vi "RecordAPP.vi"() -> ()   [LabVIEW 2022 SP3]
uses:
  <vilib>/sound2/lvsound2.llb/Sound Data Format.ctl
  <vilib>/sound2/lvsound2.llb/Sound Input Task ID.ctl
  <vilib>/Utility/miscctls.llb/LVPointTypeDef.ctl
  <vilib>/sound2/lvsound2.llb/Sound Input Read (DBL).vi
  <vilib>/sound2/lvsound2.llb/Sound Output Write (DBL Single).vi
  <vilib>/regexp/Match Regular Expression.xnode
  <vilib>/sound2/lvsound2.llb/Sound Output Write (DBL).vi
panel:
  in  "expand":bool
  out "Record":bool
  out "Play":bool
  in  "Sec.Play(K)":bool
  out "Resolution":dbl format="%.10f"
  out "Record_Graph":cluster{"x":dbl[], "y":dbl[]}(graph)
  in  "device ID":u32
  out "Record":waveform(dbl)[](graph)
  in  "stop":bool
  out "error out":errorcluster
  in  "AnalysisRecord_read(M)":bool
  in  "StartStopRecord(B)":bool
  in  "path":path
  out "VoiceData":dbl[](array[numeric])
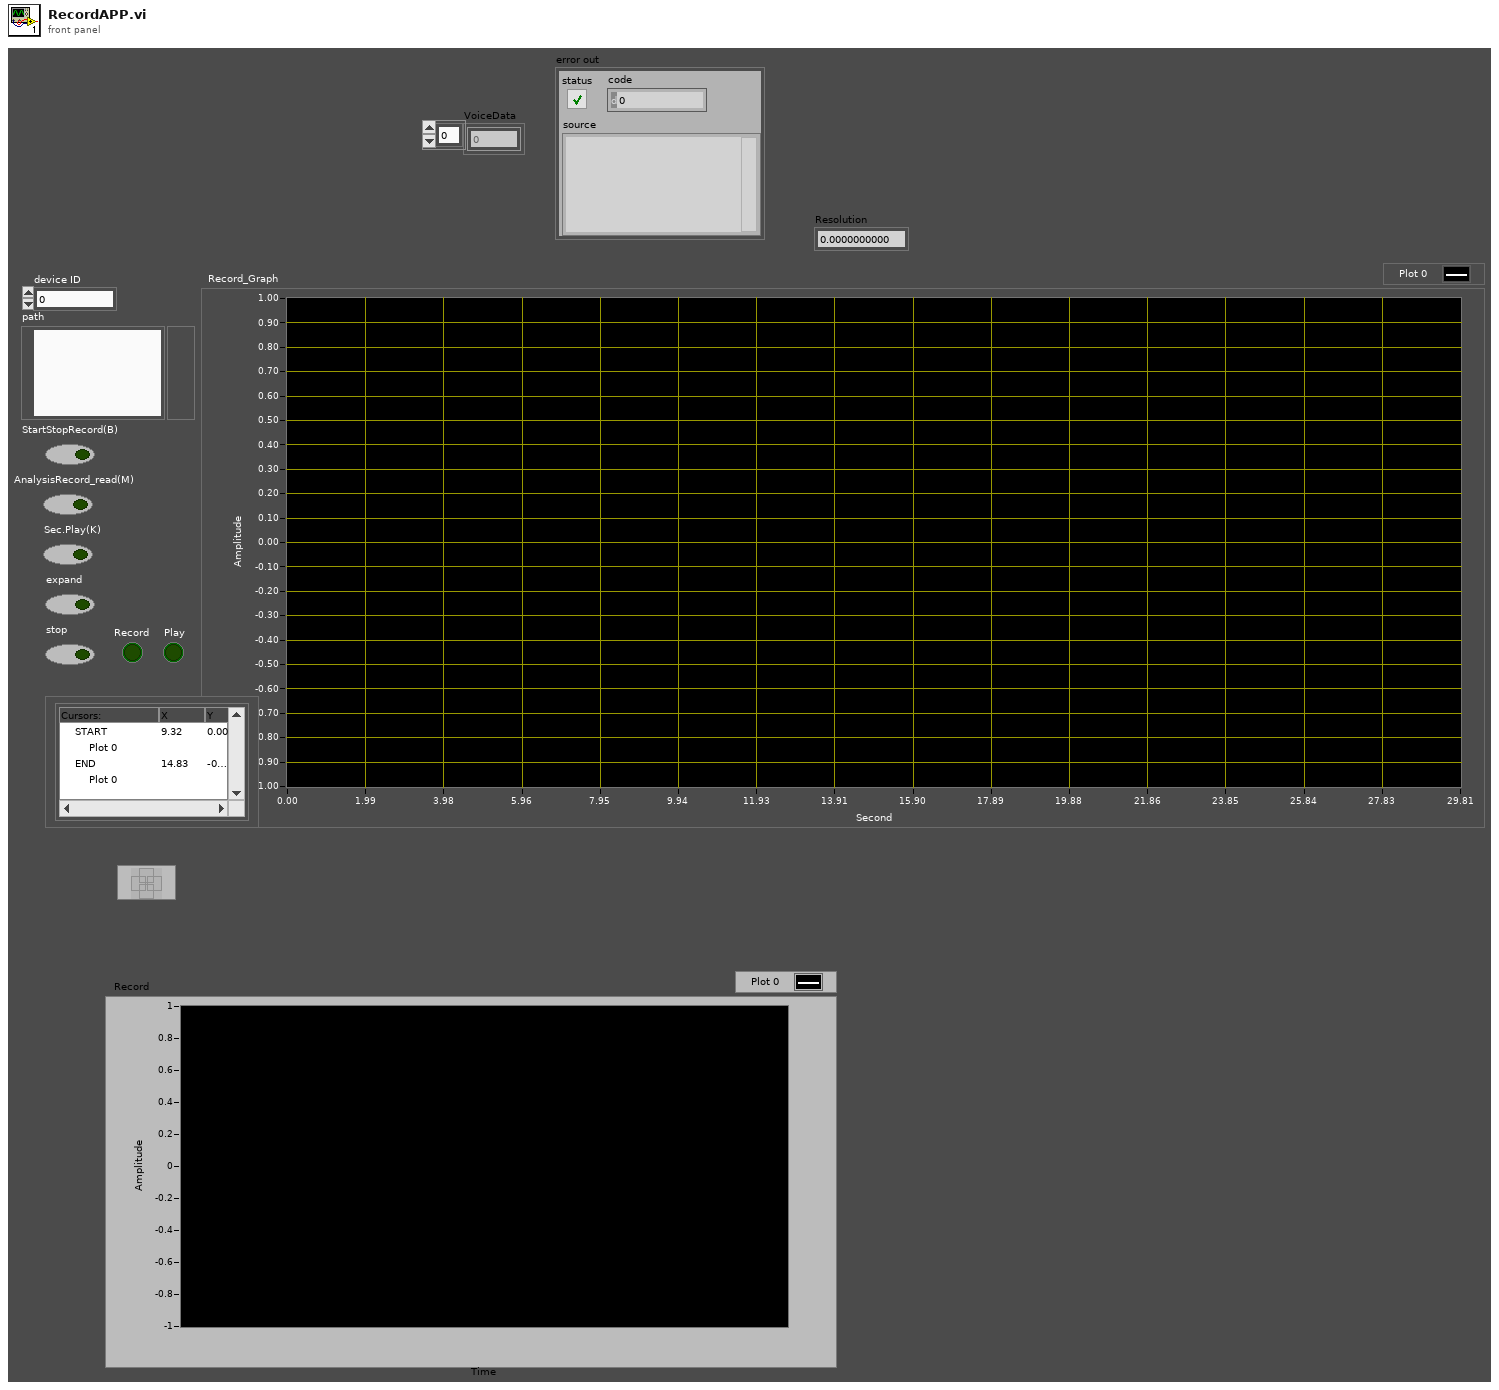
[diagram p1: front panel]
types:
  T1 = typedef "Sound Data Format.ctl" = cluster{"sample rate (S/s)":dbl, "number of channels":i32, "bits per sample":i32}
  T2 = typedef "LVPointTypeDef.ctl" = cluster{"Horizontal":i16, "Vertical":i16}
  T3 = typedef "Sound Input Task ID.ctl" = u32
  T4 = typedef "LVRectTypeDef.ctl" = cluster{"Left":i16, "Top":i16, "Right":i16, "Bottom":i16}
  T5 = typedef "Sound Output Task ID.ctl" = u32
  T6 = enum16{"open", "open or create", "create or replace", "create", "open (read-only)"}
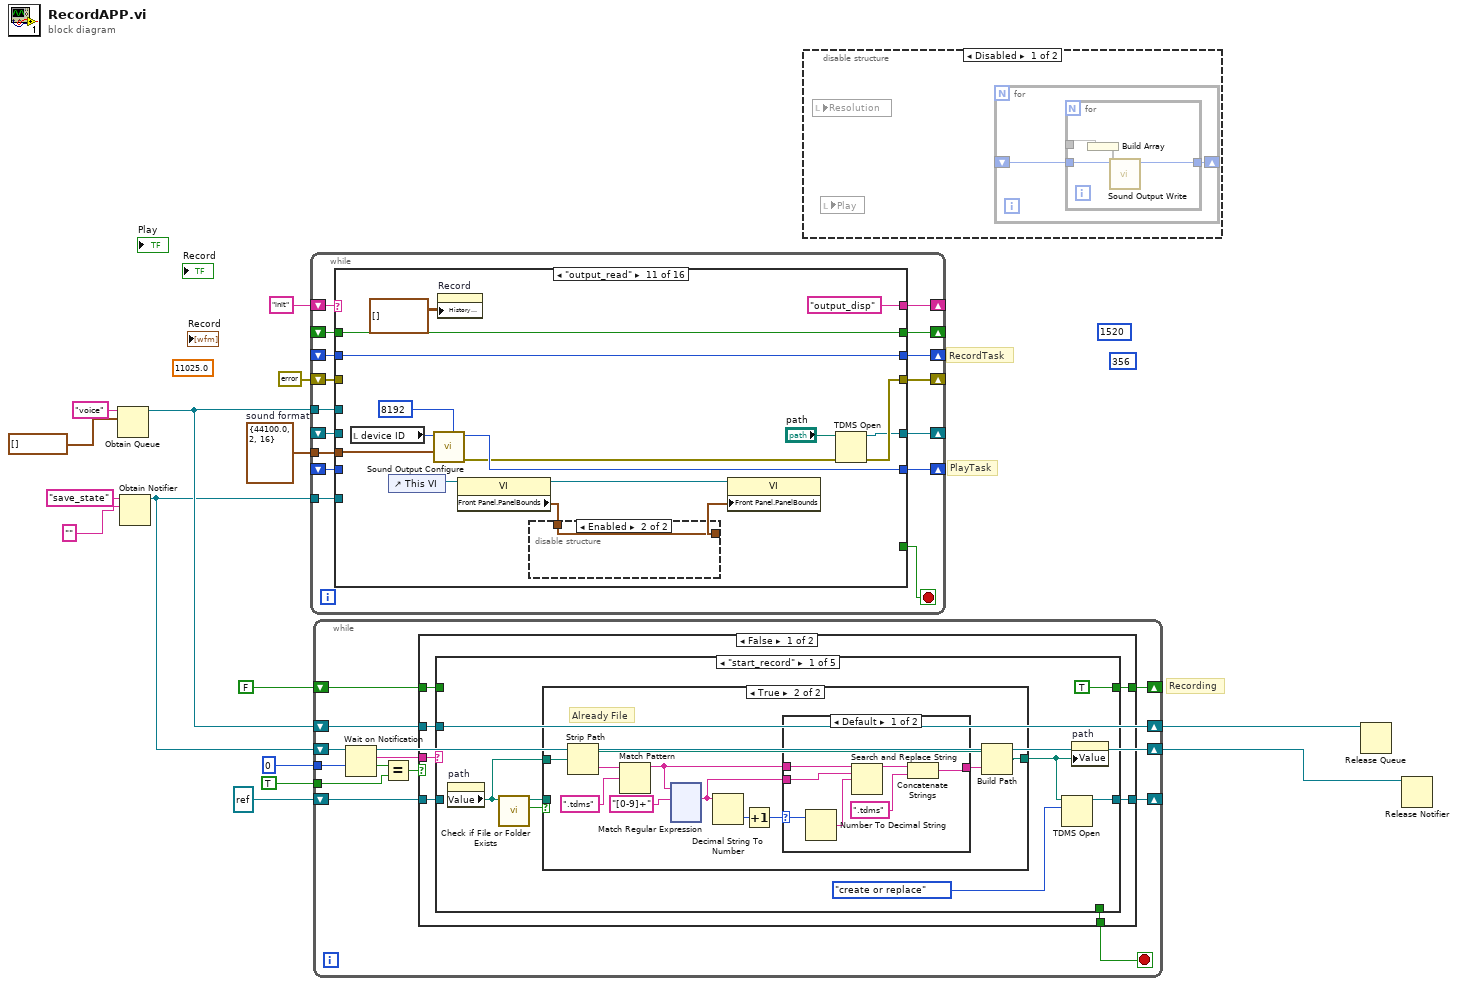
[diagram p0: block diagram]
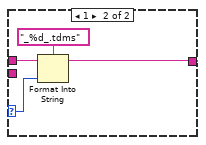
[diagram p4: hidden frame]
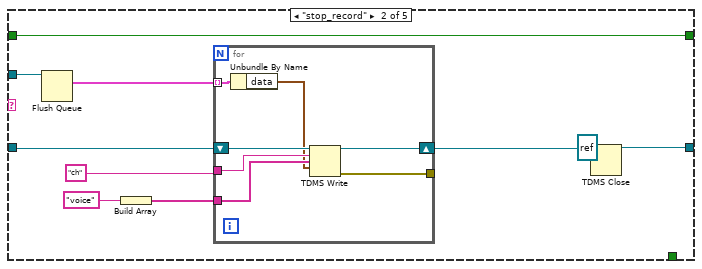
[diagram p5: hidden frame]
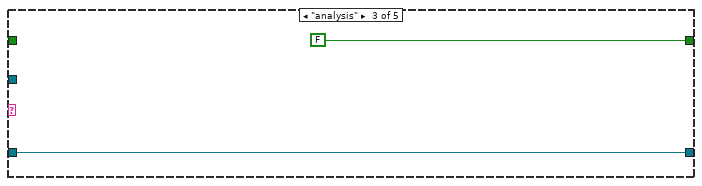
[diagram p6: hidden frame]
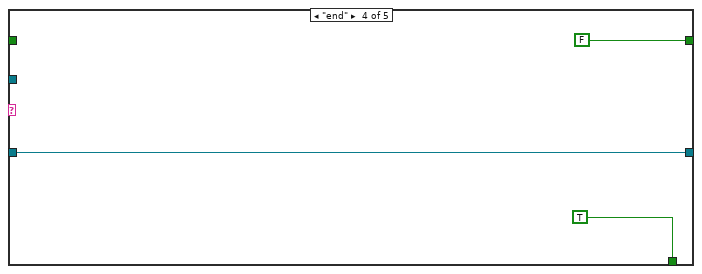
[diagram p7: hidden frame]
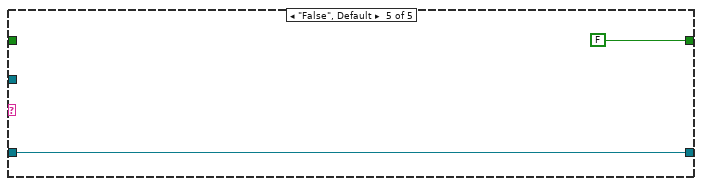
[diagram p8: hidden frame]
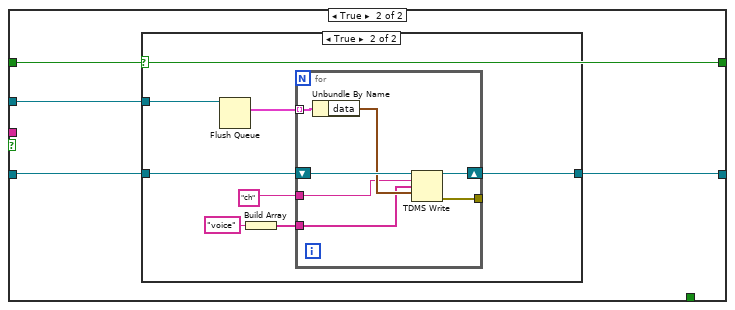
[diagram p9: hidden frame]
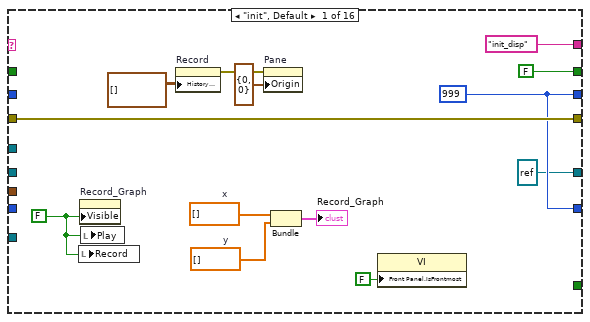
[diagram p11: hidden frame]
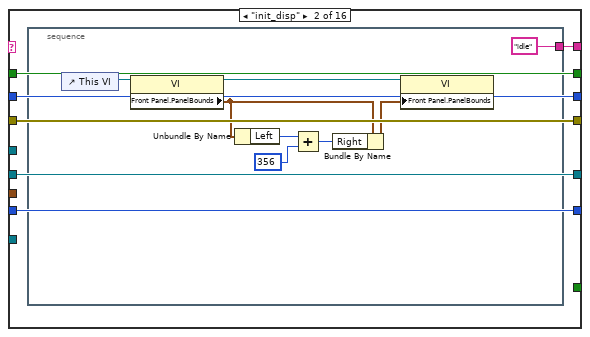
[diagram p12: hidden frame]
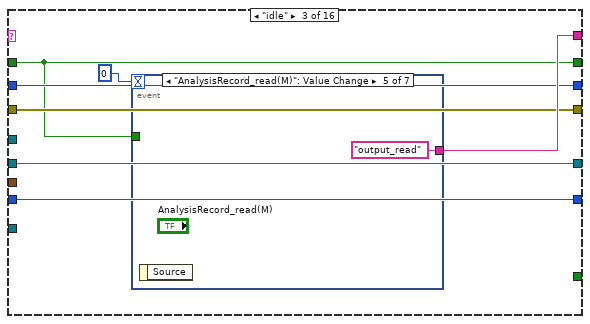
[diagram p13: hidden frame]
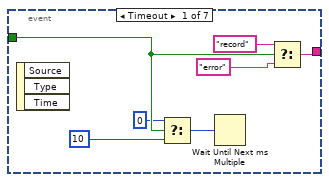
[diagram p14: hidden frame]
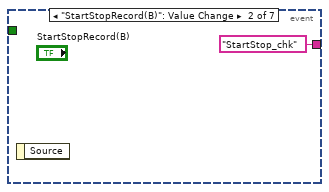
[diagram p15: hidden frame]
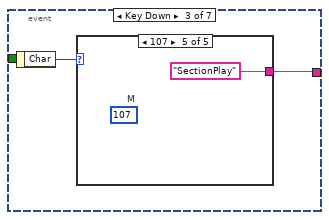
[diagram p16: hidden frame]
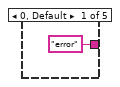
[diagram p17: hidden frame]
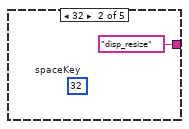
[diagram p18: hidden frame]
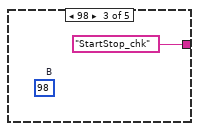
[diagram p19: hidden frame]
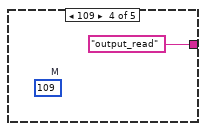
[diagram p20: hidden frame]
diagram:
  (unwired) u32 356 ("Bounds:Area Width 2")
  (unwired) u32 1520 ("Bounds:Area Width")
  (unwired) 11025.0 ("sample rate (S/s)")
  w2 = T1 {"sample rate (S/s)"=44100.0, "number of channels"=2, "bits per sample"=16}  # sound format
  # "Recording"
  # "RecordTask"
  # "PlayTask"
  n1 = Obtain Queue(name (unnamed)="voice", element data type=waveform(dbl)[] [] ("data")) -> (queue out=w11:refnum<queue>)  [unwired: 3 in, 2 out]
  n2 = Obtain Notifier(name (unnamed)="save_state", notification data type="") -> (notifier out=w7:refnum<notifier>)  [unwired: 2 in, 2 out]
  n3 = while {
    shift-right: [w30] -> _
    shift-left: "init" -> [w31]
    shift-right: [w29] -> _
    shift-left: _ -> [w28]
    shift-right: [w27] -> _
    shift-left: errorcluster {"status"=FALSE, "code"=0, "source"=""} ("error out") -> [w26]
    shift-right: [w25] -> _
    shift-left: _ -> [w24]
    tunnel: w11 -> [w23]
    tunnel: w7 -> [w22]
    tunnel: w2 -> [w20]
    shift-right: [w19] -> _
    shift-left: _ -> [w18]
    shift-right: [w17] -> _
    shift-left: _ -> [w16]
    stop <- w21 stop-if-true
    n4 = case shown="\"output_read\"" w31 {
      tunnel: ["init_disp" w50 w64 w98 w107 w114 w133 "error" "idle" "idle" "output_disp" "output_disp2" w240 w293 "idle" "end"] -> w30
      tunnel: [w40 w49 w63 w100 w106 w113 w132 w157 w173 T3 999 ("task ID out") w204 w233 w239 w292 w323 w332] -> w29
      tunnel: w28 -> [_ w49 w63 w100 w106 w113 w132 _ w172 w188 w204 w233 w239 w292 w323 w332]
      tunnel: [w43 w48 w62 w96 w105 w112 w131 w156 w162 w176 w201 w232 w238 w291 w320 w331] -> w27
      tunnel: w26 -> [w43 w48 w62 w96 w105 w112 w131 w147 w171 w185 _ w232 w238 w291 w322 w331]
      tunnel: [FALSE w47 w61 w95 w104 w111 w130 TRUE w174 FALSE w203 w231 w237 w290 w321 w330] -> w25
      tunnel: w24 -> [_ w47 w61 w95 w104 w111 w130 _ w174 _ w203 w231 w237 w290 w321 w330]
      tunnel: w23 -> [_ _ _ _ _ _ _ _ w170 _ _ _ _ _ _ _]
      tunnel: w22 -> [_ _ _ _ _ _ _ w153 _ w181 _ w224 _ _ _ w328]
      tunnel: [_ _ _ _ _ _ _ _ _ _ _ _ _ _ _ TRUE] -> w21
      tunnel: w20 -> [_ _ _ _ _ _ _ w158 _ _ w198 _ _ _ _ _]
      tunnel: [refnum<k34> refnum ("tdms file out") w46 w60 w93 w103 w110 w129 w151 w166 w180 w200 refnum<k34> refnum ("tdms file out") w236 w289 w319 w326] -> w19
      tunnel: w18 -> [_ w46 w60 w93 w103 w110 w129 w151 w166 w180 _ w230 w236 w289 w319 w326]
      tunnel: [w40 w45 w59 w92 w102 w109 w128 w150 w165 w179 w196 w217 w235 w287 w318 w325] -> w17
      tunnel: w16 -> [_ w45 w59 w92 w102 w109 w128 w150 w165 w179 _ w217 w235 w288 w318 w325]
      frame "init", Default {
        w35 = dbl[] []  # y
        w36 = dbl[] []  # x
        w38 = FALSE ("Visible")
        w40 = T3 999 ("task ID out")
        n5 = local write "Record"(w38) -> ()
        n6 = property on="Record_Graph" class="XYGraph (strict)"("Visible"=w38) -> ()  [unwired: 2 in, 2 out]
        n7 = local write "Play"(w38) -> ()
        n8 = property on="Record" class="WFChart (strict)"("History Data"=waveform(dbl)[][] []) -> (error out=w34:errorcluster)  [unwired: 2 in, 1 out]
        n9 = property on="Pane" class="Pane"(error in=w34, "Origin"=T2 {"Horizontal"=0, "Vertical"=0}) -> ()  [unwired: 1 in, 2 out]
        n10 = Bundle("x"=w36, "y"=w35) -> (→"Record_Graph":cluster{"x":dbl[], "y":dbl[]})  [unwired: 1 in]
        n11 = property class="VI"("Front Panel.IsFrontmost"=FALSE ("Front Panel Window:Is Frontmost")) -> ()  [unwired: 2 in, 2 out]
      }
      frame "init_disp" {
        n12 = stacked-sequence {
          tunnel: ["idle"] -> w50
          frame #0 {
            n13 = control-ref of="This VI"() -> (w57:refnum<vi>)
            n14 = property class="VI"(reference=w57) -> (reference out=w56:refnum<vi>, "Front Panel.PanelBounds"=w53:T4)  [unwired: 1 in, 1 out]
            n15 = Unbundle By Name(w53) -> ("Left"=w55:i16)
            n16 = Add(x=w55, y=u32 356 ("Bounds:Area Width 2")) -> (x+y=w51:u32)
            n17 = Bundle By Name(cluster=w53, "Right"=w51) -> (w52:T4)
            n18 = property class="VI"(reference=w56, "Front Panel.PanelBounds"=w52) -> ()  [unwired: 1 in, 2 out]
          }
        }
      }
      frame "idle" {
        n19 = event shown="[4] \"AnalysisRecord_read(M)\": Value Change" {
          selector: _ -> [_ _ _ _ _ _ _]
          dyn-events: _ -> [_ _ _ _ _ _ _]
          timeout: 0 -> [_ _ _ _ _ _ _]
          tunnel: [w71 "StartStop_chk" w74 "end" "output_read" ("t") "SectionPlay" ("t") "expand" ("t")] -> w64
          tunnel: w61 -> [w68 _ _ _ _ _ _]
          event Timeout {
            n20 = event-data() -> ()  [unwired: 1 in, 3 out]
            n21 = Select(t=u32 0, s=w68, f=u32 10 ("millisecond multiple")) -> (s? t:f=w69:u32)
            n22 = Wait Until Next ms Multiple(millisecond multiple=w69) -> ()  [unwired: 1 out]
            n23 = Select(t="record", s=w68, f="error") -> (s? t:f=w71:string)
          }
          event "StartStopRecord(B)": Value Change {
            n24 = event-data() -> ()  [unwired: 1 in, 1 out]
          }
          event Key Down {
            n25 = event-data() -> ("Char"=w75:i16)  [unwired: 1 in]
            n26 = case shown="107" w75 {
              tunnel: ["error" ("t") "disp_resize" ("t") "StartStop_chk" ("t") "output_read" ("t") "SectionPlay" ("t")] -> w74
              frame 0, Default {
              }
              frame 32 {
                (unwired) i16 32  # spaceKey
              }
              frame 98 {
                (unwired) i16 98  # B
              }
              frame 109 {
                (unwired) i16 109  # M
              }
              frame 107 {
                (unwired) i16 107  # M
              }
            }
          }
          event "stop": Value Change {
            n27 = event-data() -> ()  [unwired: 1 in, 1 out]
          }
          event "AnalysisRecord_read(M)": Value Change {
            n28 = event-data() -> ()  [unwired: 1 in, 1 out]
          }
          event "Sec.Play(K)": Value Change {
            n29 = event-data() -> ()  [unwired: 1 in, 1 out]
          }
          event "expand": Value Change {
            n30 = event-data() -> ()  [unwired: 1 in, 1 out]
          }
        }
      }
      frame "StartStop_chk" {
        n31 = control-ref of="This VI"() -> (w91:refnum<vi>)
        n32 = Equal?(x=w100, y=T3 999) -> (x = y?=w94:bool)
        n33 = property class="VI"(reference=w91) -> (reference out=w90:refnum<vi>, "Front Panel.PanelBounds"=w87:T4)  [unwired: 1 in, 1 out]
        n34 = Unbundle By Name(w87) -> ("Left"=w89:i16)
        n35 = Add(x=w89, y=u32 356 ("Bounds:Area Width 2")) -> (x+y=w85:u32)
        n36 = Bundle By Name(cluster=w87, "Right"=w85) -> (w86:T4)
        n37 = property class="VI"(reference=w90, "Front Panel.PanelBounds"=w86) -> ()  [unwired: 1 in, 2 out]
        n38 = Select(t="start", s=w94, f="stop") -> (s? t:f=w98:string)
      }
      frame "xxxxxxxxxxx" {
        n39 = stacked-sequence {
          tunnel: ["idle"] -> w107
          frame #0 {
          }
        }
      }
      frame "disp_resize" {
        n40 = stacked-sequence {
          tunnel: ["idle"] -> w114
          frame #0 {
            w117 = u32 356 ("Bounds:Area Width 2")
            n41 = property class="VI"() -> (reference out=w126:refnum<vi>, "Front Panel.PanelBounds"=w125:T4)  [unwired: 2 in, 1 out]
            n42 = Unbundle By Name(w125) -> ("Right"=w123:i16, "Left"=w118:i16)
            n43 = Subtract(x=w123, y=w118) -> (x-y=w122:i16)
            n44 = Less Or Equal?(x=w122, y=w117) -> (x <= y?=w120:bool)
            n45 = Add(x=w118, y=w117) -> (x+y=w116:u32)
            n46 = Add(x=w118, y=u32 1520 ("Bounds:Area Width")) -> (x+y=w115:u32)
            n47 = Select(t=w115, s=w120, f=w116) -> (s? t:f=w121:u32)
            n48 = Bundle By Name(cluster=w125, "Right"=w121) -> (w124:T4)
            n49 = property class="VI"(reference=w126, "Front Panel.PanelBounds"=w124) -> ()  [unwired: 1 in, 2 out]
          }
        }
      }
      frame "expand" {
        n50 = stacked-sequence {
          tunnel: ["idle"] -> w133
          frame #0 {
            w140 = 10
            w141 = u32 1  # y
            w142 = u32 0  # x
            n51 = property on="Record_Graph" class="XYGraph (strict)"("Active Cursor"=w142, "Active Cursor"=w141) -> ("Cursor.Cursor X"=w135:dbl, "Cursor.Cursor X"=w136:dbl)  [unwired: 2 in, 2 out]
            n52 = Subtract(x=w136, y=w135) -> (x-y=w134:dbl)
            n53 = Divide(x=w134, y=w140) -> (x/y=w139:dbl)
            n54 = for {
              N: w140 -> [_]
              tunnel: w139 -> [w146]
              tunnel: [w144] -> w138 mode=indexing
              shift-right: [w144] -> _
              shift-left: w135 -> [w145]
              n55 = Add(x=w145, y=w146) -> (x+y=w144:dbl)
            }
            n56 = Build Array (concatenate)(w135, w138) -> (w137:dbl[])
            n57 = property on="Record_Graph" class="XYGraph (strict)"("XScale.RngStart"=w135, "XScale.Minimum"=w135, "XScale.Maximum"=w136, "XScale.Increment"=w139, "XScale.MarkerVals[]"=w137) -> ()  [unwired: 2 in, 2 out]
          }
        }
      }
      frame "start" {
        n58 = property on="Record_Graph" class="XYGraph (strict)"("Visible"=FALSE) -> ()  [unwired: 2 in, 2 out]
        n59 = local write "Record"(TRUE ("Record")) -> ()
        n60 = Send Notification(notification="start_record", notifier=w153, error in (no error)=w147) -> (error out=w152:errorcluster)  [unwired: 1 out]
        n61 = call <vilib>:"Sound Input Configure.vi"("number of samples/ch"=8192, "error in (no error)"=w152, "sound format"=w158, "device ID"="device ID") -> ("error out"=w156:errorcluster, "task ID"=w157:T3)  [unwired: 6 in]
      }
      frame "record" {
        n62 = Quotient & Remainder(x=8192 ("number of samples/ch"), y=2) -> (floor(x/y)=w167:i32)  [unwired: 1 out]
        n63 = call-poly <vilib>:"Sound Input Read.vi"("number of samples/ch"=w167, "error in (no error)"=w171, "task ID"=w172) -> ("error out"=w163:errorcluster, "data"=w164:waveform(dbl)[], "task ID out"=w173:T3)  [unwired: 6 in]
        n64 = Enqueue Element(queue=w170, element=w164, error in (no error)=w163) -> (error out=w162:errorcluster)  [unwired: 1 in, 2 out]
      }
      frame "stop" {
        n65 = call <vilib>:"Sound Input Stop.vi"("error in (no error)"=w185, "task ID"=w188) -> ("error out"=w186:errorcluster, "task ID out"=w187:T3)  [unwired: 8 in]
        n66 = call <vilib>:"Sound Input Clear.vi"("error in (no error)"=w186, "task ID"=w187) -> ("error out"=w182:errorcluster)  [unwired: 9 in]
        n67 = Send Notification(notification="stop_record", notifier=w181, error in (no error)=w182) -> (error out=w176:errorcluster)  [unwired: 1 out]
        n68 = local write "Record"(FALSE ("Record")) -> ()
      }
      frame "output_read" {
        n69 = local read "device ID"() -> (w199:u32)
        n70 = control-ref of="This VI"() -> (w193:refnum<vi>)
        n71 = call <vilib>:"Sound Output Configure.vi"("number of samples/ch"=8192, "sound format"=w198, "device ID"=w199) -> ("error out"=w194:errorcluster, "task ID"=w196:T5)  [unwired: 7 in]
        n72 = property on="Record" class="WFChart (strict)"("History Data"=waveform(dbl)[][] []) -> ()  [unwired: 2 in, 2 out]
        n73 = property class="VI"(reference=w193) -> (reference out=w192:refnum<vi>, "Front Panel.PanelBounds"=w191:T4)  [unwired: 1 in, 1 out]
        n74 = disable-structure shown="Enabled" {
          disable-tunnel: w191 -> [w209 w211]
          disable-tunnel: [w208 w211] -> w190
          frame Disabled {
            n75 = Unbundle By Name(w209) -> ("Left"=w210:i16)
            n76 = Add(x=w210, y=u32 1520 ("Bounds:Area Width")) -> (x+y=w207:u32)
            n77 = Bundle By Name(cluster=w209, "Right"=w207) -> (w208:T4)
          }
          frame Enabled {
          }
        }
        n78 = property class="VI"(reference=w192, "Front Panel.PanelBounds"=w190) -> ()  [unwired: 1 in, 2 out]
        n79 = TDMS Open(8:w194, 11:"path") -> (0:w201:errorcluster, 3:w200:refnum<k34>)  [unwired: 5 in]
      }
      frame "output_disp" {
        w215 = "voice" ("group name in")
        n80 = Build Array(w215) -> (w227:string[])
        n81 = TDMS Read(0:w230, 5:"ch" ("group name in"), 7:w227, 12:waveform(dbl)[] [] ("data")) -> (4:w221:refnum<k34>, 6:w216:string, 10:w226:waveform(dbl)[], 15:w223:errorcluster)  [unwired: 4 in, 2 out]
        n82 = Send Notification(notification="analysis", notifier=w224, error in (no error)=w223) -> (error out=w220:errorcluster)  [unwired: 1 out]
        n83 = local write "Record"(w226) -> ()
        n84 = TDMS Get Properties(5:0.0, 7:"wf_increment" ("channel name"), 8:w220, 9:w215, 10:w216, 11:w221) -> (0:w213:errorcluster, 3:w214:refnum<k34>, 4:→"Resolution":dbl)  [unwired: 3 out]
        n85 = TDMS Close(8:w213, 11:w214) -> ()  [unwired: 2 out]
      }
      frame "output_disp2" {
        n86 = stacked-sequence {
          seq-local: [_ w243 _ _] -> [_ _ w256 w273]
          seq-local: [_ w242 _ _] -> [_ _ _ w275]
          tunnel: [_ "idle" _ _] -> w240
          frame #0 {
            n87 = property on="Record_Graph" class="XYGraph (strict)"("Visible"=TRUE) -> ()  [unwired: 2 in, 2 out]
          }
          frame #1 {
            n88 = local read "Record"() -> (w248:waveform(dbl)[])
            n89 = local read "Resolution"() -> (w246:dbl)
            n90 = for {
              tunnel: w248 -> [w254] mode=indexing
              tunnel: [w253] -> w242 mode=concatenating
              n91 = Unbundle By Name(w254) -> ("Y"=w253:dbl[])
            }
            "VoiceData" <- w242
            n92 = Array Size(array=w242) -> (size(s)=w244:i32)
            n93 = for {
              N: w244 -> [_]
              tunnel: w246 -> [w252]
              tunnel: [w250] -> w243 mode=indexing
              i -> [w251]
              n94 = Multiply(x=w252, y=w251) -> (x*y=w250:dbl)
            }
            n95 = Bundle By Name(cluster=cluster{"x":dbl[], "y":dbl[]} {"x"=[], "y"=[]} ("output cluster"), "x"=w243, "y"=w242) -> (w245:cluster{"x":dbl[], "y":dbl[]})
            n96 = local write "Record_Graph"(w245) -> ()
          }
          frame #2 {
            w260 = 15
            n97 = Array Size(array=w256) -> (size(s)=w258:i32)
            n98 = Decrement(x=w258) -> (x-1=w255:i32)
            n99 = Index Array(array=w256, index #2=w255) -> (element #1=w259:dbl, element #2=w257:dbl)  [unwired: 1 in]
            n100 = Subtract(x=w257, y=w259) -> (x-y=w261:dbl)
            n101 = Divide(x=w261, y=w260) -> (x/y=w264:dbl)
            n102 = for {
              N: w260 -> [_]
              tunnel: w264 -> [w267]
              tunnel: [w265] -> w263 mode=indexing
              shift-right: [w265] -> _
              shift-left: w259 -> [w266]
              n103 = Add(x=w266, y=w267) -> (x+y=w265:dbl)
            }
            n104 = Build Array (concatenate)(w259, w263) -> (w262:dbl[])
            n105 = property on="Record_Graph" class="XYGraph (strict)"("XScale.RngStart"=w259, "XScale.Minimum"=w259, "XScale.Maximum"=w257, "XScale.Increment"=w264, "XScale.MarkerVals[]"=w262) -> ()  [unwired: 2 in, 2 out]
          }
          frame #3 {
            w282 = 0.5  # sec
            w286 = 0.5  # Hz
            n106 = Greater Or Equal?(x=w275, y=w286) -> (x >= y?=w285:bool[])
            n107 = Search 1D Array(1D array=w285, element=TRUE) -> (index of element=w283:i32)  [unwired: 1 in]
            n108 = Index Array(array=w273, index=w283) -> (element=w281:dbl)
            n109 = Subtract(x=w281, y=w282) -> (x-y=w280:dbl)
            n110 = Array Size(array=w273) -> (size(s)=w272:i32)
            n111 = Greater Or Equal?(x=w273, y=w280) -> (x >= y?=w278:bool[])
            n112 = Search 1D Array(1D array=w278, element=TRUE) -> (index of element=w270:i32)  [unwired: 1 in]
            n113 = Subtract(x=w272, y=500 ("x")) -> (x-y=w271:i32)
            n114 = Index Array(array=w273, index #1=w271, index #2=w270) -> (element #1=w276:dbl, element #2=w269:dbl)
            n115 = property on="Record_Graph" class="XYGraph (strict)"("Active Cursor"=u32 1, "Cursor.Cursor X"=w276, "Active Cursor"=u32 0, "Cursor.Cursor X"=w269) -> ()  [unwired: 2 in, 2 out]
          }
        }
      }
      frame "SectionPlay" {
        n116 = stacked-sequence {
          tunnel: [_ "idle" _] -> w293
          tunnel: w288 -> [_ w299 _]
          tunnel: [_ w297 _] -> w287
          frame #0 {
            n117 = local write "Play"(TRUE ("Play")) -> ()
          }
          frame #1 {
            w307 = u32 1  # y
            w308 = u32 0  # x
            n118 = local read "Record_Graph"() -> (w309:cluster{"x":dbl[], "y":dbl[]})
            n119 = property on="Record_Graph" class="XYGraph (strict)"("Active Cursor"=w308, "Active Cursor"=w307) -> ("Cursor.Cursor X"=w306:dbl, "Cursor.Cursor X"=w304:dbl)  [unwired: 2 in, 2 out]
            n120 = Unbundle By Name(w309) -> ("y"=w303:dbl[], "x"=w305:dbl[])
            n121 = Search 1D Array(1D array=w305, element=w306) -> (index of element=w301:i32)  [unwired: 1 in]
            n122 = Search 1D Array(1D array=w305, element=w304) -> (index of element=w302:i32)  [unwired: 1 in]
            n123 = Subtract(x=w302, y=w301) -> (x-y=w300:i32)
            n124 = Array Subset(array=w303, index=w301, length=w300) -> (w296:dbl[])
            n125 = for {
              N: 1 -> [_]
              tunnel: w299 -> [w315]
              tunnel: [w314] -> w297
              shift-right: [w312] -> _
              shift-left: dbl[] [0.0] -> [w312]
              tunnel: w296 -> [w311]
              tunnel: [w313] -> _
              n126 = Replace Array Subset(array=w312, new element=w312) -> ()  [unwired: 1 in, 1 out]
              n127 = call-poly <vilib>:"Sound Output Write.vi"("data"=w311, "task ID"=w315) -> ("error out"=w313:errorcluster, "task ID out"=w314:T5)  [unwired: 8 in]
            }
          }
          frame #2 {
            n128 = flat-sequence {
              frame #0 {
                n129 = Wait (ms)(milliseconds to wait=u32 50) -> ()  [unwired: 1 out]
              }
              frame #1 {
                n130 = local write "Play"(FALSE ("Play")) -> ()
              }
            }
          }
        }
      }
      frame "error" {
        n131 = call <vilib>:"Clear Errors.vi"("error in (no error)"=w322) -> ("error out"=w320:errorcluster)  [unwired: 5 in, 1 out]
        "error out" <- w322
      }
      frame "end" {
        n132 = Send Notification(notification="end", notifier=w328) -> ()  [unwired: 1 in, 2 out]
      }
    }
  }
  n133 = while {
    shift-right: [w341] -> _
    shift-left: FALSE -> [w340]
    tunnel: TRUE ("y") -> [w344]
    shift-right: [w339] -> _
    shift-left: refnum<k34> refnum ("tdms file out") -> [w337]
    shift-right: [w335] -> w4
    shift-left: w11 -> [w335]
    shift-right: [w336] -> w3
    shift-left: w7 -> [w346]
    tunnel: 0 ("timeout in ms (-1)") -> [w334]
    stop <- w338 stop-if-true
    n134 = Wait on Notification(notifier=w346, timeout in ms (-1)=w334) -> (notifier out=w336:refnum<notifier>, notification=w342:string, timed out?=w345:bool)  [unwired: 2 in, 1 out]
    n135 = Equal?(x=w345, y=w344) -> (x = y?=w343:bool)
    n136 = case shown="False" w343 {
      tunnel: w335 -> [w348 w526]
      tunnel: w342 -> [w353 _]
      tunnel: [w352 w527] -> w341
      tunnel: w340 -> [w351 w527]
      tunnel: [w350 w524] -> w339
      tunnel: w337 -> [w349 w525]
      tunnel: [w347 _] -> w338
      frame False {
        n137 = case shown="\"start_record\"" w353 {
          tunnel: [TRUE w509 FALSE FALSE FALSE] -> w352
          tunnel: w351 -> [_ w509 _ _ _]
          tunnel: [w358 refnum<k34> refnum ("tdms file out") w517 w520 w522] -> w350
          tunnel: w349 -> [_ w504 w517 w520 w522]
          tunnel: w348 -> [_ w505 _ _ _]
          tunnel: [_ _ _ TRUE _] -> w347
          frame "start_record" {
            n138 = property on="path" class="Path"() -> ("Value"=w355:path)  [unwired: 2 in, 2 out]
            n139 = call <vilib>:"Check if File or Folder Exists.vi"("path"=w355) -> ("file or folder exists?"=w357:bool, "dup path"=w356:path)  [unwired: 8 in, 1 out]
            n140 = case shown="True" w357 {
              tunnel: w356 -> [_ _]
              tunnel: w355 -> [w361 w363]
              tunnel: [w361 w362] -> w354
              frame False {
              }
              frame True {
                # "Already File"
                n141 = Strip Path(path=w363) -> (stripped path=w371:path, name=w366:string)
                n142 = Match Pattern(string=w366, regular expression=".tdms") -> (before substring=w369:string)  [unwired: 1 in, 3 out]
                n143 = xnode "Match Regular Expression"("input string"=w369, "regular expression"="[0-9]+") -> ("whole match"=w370:string)  [unwired: 4 in, 4 out]
                n144 = Decimal String To Number(string=w370) -> (number=w367:i32)  [unwired: 2 in, 1 out]
                n145 = Increment(x=w367) -> (x+1=w368:i32)
                n146 = case shown="Default" w368 {
                  selector: w368 -> [w377 w381]
                  tunnel: w369 -> [w379 w382]
                  tunnel: [w374 w380] -> w372
                  tunnel: w370 -> [w378 _]
                  frame Default {
                    n147 = Number To Decimal String(number=w377) -> (decimal integer string=w376:string)  [unwired: 1 in]
                    n148 = Search and Replace String(input string=w379, search string=w378, replace string=w376) -> (result string=w375:string)  [unwired: 5 in, 3 out]
                    n149 = Concatenate Strings(w375, ".tdms" ("string")) -> (w374:string)
                  }
                  frame 1 {
                    n150 = Format Into String(format string="_%d_.tdms", initial string=w382, w381) -> (resulting string=w380:string)  [unwired: 1 in, 1 out]
                  }
                }
                n151 = Build Path(base path=w371, name or relative path=w372) -> (appended path=w362:path)
              }
            }
            n152 = TDMS Open(10:T6."create or replace" ("operation (0:open)"), 11:w354) -> (3:w358:refnum<k34>)  [unwired: 5 in, 1 out]
            n153 = property on="path" class="Path"("Value"=w354) -> ()  [unwired: 2 in, 2 out]
          }
          frame "stop_record" {
            n154 = Flush Queue(queue=w505) -> (remaining elements=w507:cluster{"data":waveform(dbl)[]}[])  [unwired: 1 in, 2 out]
            n155 = Build Array("voice") -> (w501:string[])
            n156 = for {
              tunnel: w507 -> [w514] mode=indexing
              shift-right: [w515] -> w503
              shift-left: w504 -> [w516]
              tunnel: "ch" -> [w513]
              tunnel: w501 -> [w512]
              tunnel: [w510] -> _
              n157 = Unbundle By Name(w514) -> ("data"=w511:waveform(dbl)[])
              n158 = TDMS Write(0:w516, 5:w513, 7:w512, 9:w511) -> (4:w515:refnum<k34>, 15:w510:errorcluster)  [unwired: 2 in, 2 out]
            }
            n159 = TDMS Close(11:w503) -> ()  [unwired: 1 in, 2 out]
          }
          frame "analysis" {
          }
          frame "end" {
          }
          frame "False", Default {
          }
        }
      }
      frame True {
        n160 = case shown="True" w527 {
          tunnel: w526 -> [_ w535]
          tunnel: w525 -> [w528 w533]
          tunnel: [w528 w532] -> w524
          frame False {
          }
          frame True {
            n161 = Flush Queue(queue=w535) -> (remaining elements=w534:cluster{"data":waveform(dbl)[]}[])  [unwired: 1 in, 2 out]
            n162 = Build Array("voice") -> (w529:string[])
            n163 = for {
              tunnel: w534 -> [w540] mode=indexing
              shift-right: [w541] -> w532
              shift-left: w533 -> [w542]
              tunnel: "ch" -> [w538]
              tunnel: w529 -> [w537]
              tunnel: [w536] -> _
              n164 = Unbundle By Name(w540) -> ("data"=w539:waveform(dbl)[])
              n165 = TDMS Write(0:w542, 5:w538, 7:w537, 9:w539) -> (4:w541:refnum<k34>, 15:w536:errorcluster)  [unwired: 2 in, 2 out]
            }
          }
        }
      }
    }
  }
  n166 = disable-structure shown="Disabled" {
    frame Disabled {
      n167 = local read "Resolution"() -> ()  [unwired: 1 in]
      n168 = local read "Play"() -> ()  [unwired: 1 in]
      n169 = for {
        shift-right: [w543] -> _
        shift-left: _ -> [w544]
        n170 = for {
          tunnel: w544 -> [w548]
          tunnel: _ -> [w546]
          tunnel: [w547] -> w543
          n171 = Build Array(w546) -> (w545:void[])
          n172 = call-poly <vilib>:"Sound Output Write.vi"("data"=w545, "task ID"=w548) -> ("task ID out"=w547:T5)  [unwired: 8 in, 1 out]
        }
      }
    }
    frame Enabled {
    }
  }
  n173 = Release Queue(queue=w4) -> ()  [unwired: 2 in, 3 out]
  n174 = Release Notifier(notifier=w3) -> ()  [unwired: 2 in, 3 out]
